vi "CreateInputTunnels.vi"(5 "controlling":bool, 6 "error in":errorcluster, 9 "Loop in":refnum<class "Loop.lvclass">) -> (0 "error out":errorcluster, 3 "Loop out":refnum<class "Loop.lvclass">, 4 "createTunnels":string)   [LabVIEW 2014, in "Raspberry Pi Compatible Compiler for LabVIEW.lvlib" / "Loop.lvclass"]
uses:
  Loop.lvclass
  Python/Parsing/ClassTypeTD.ctl
  Python/Parsing/ListTypesTD.ctl
  LoopTunnel/LoopTunnel.lvclass/LoopTunnel.ctl
  Tunnel/Tunnel.lvclass/Tunnel.ctl
  Terminal/Terminal.lvclass
  Python/Parsing/Python Functions.lvlib
  LoopTunnel/LoopTunnel.lvclass
  Tunnel/Tunnel.lvclass
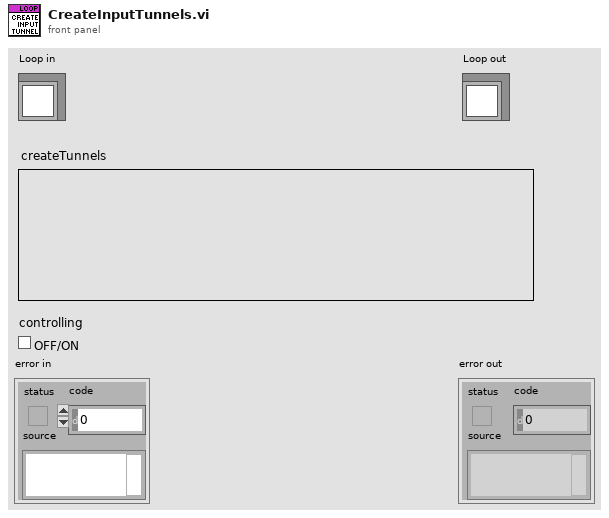
[diagram p1: front panel]
types:
  T1 = typedef "Raspberry Pi Compatible Compiler for LabVIEW.lvlib/Python Functions.lvlib/ListTypesTD.ctl" = enum16{"list", "tuple", "parameter list", "output list", "return values"}
  T2 = typedef "Raspberry Pi Compatible Compiler for LabVIEW.lvlib/Python Functions.lvlib/ClassTypeTD.ctl" = enum16{"class", "function"}
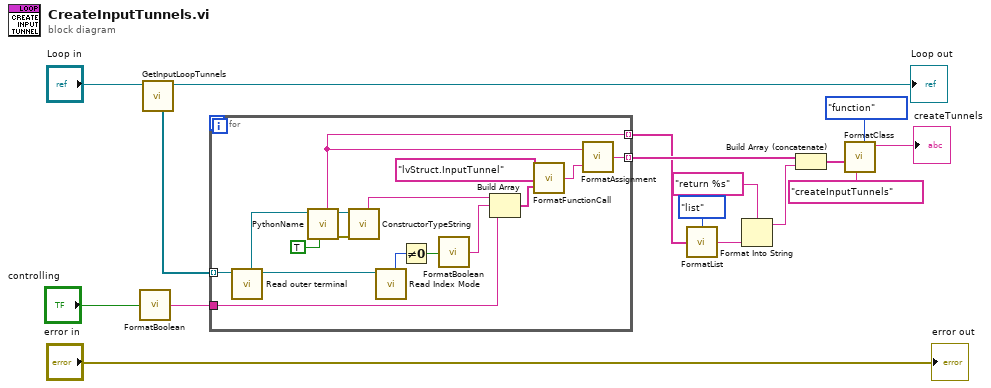
[diagram p0: block diagram]
diagram:
  n1 = call "FormatBoolean.vi"("value"="controlling") -> ("python object"=w7:string)
  n2 = call-dynamic "GetInputLoopTunnels.vi"("Loop in"="Loop in") -> ("Loop out"=→"Loop out":refnum<class "Loop.lvclass">, "tunnels"=w11:refnum<class "LoopTunnel.lvclass">[])  [unwired: 6 in, 1 out]
  n3 = for {
    tunnel: w11 -> [w30] mode=indexing
    tunnel: [w25] -> w10 mode=indexing
    tunnel: w7 -> [w19]
    tunnel: [w17] -> w6 mode=indexing
    n4 = call "Read outer terminal.vi"("Tunnel in"=w30) -> ("Tunnel out"=w31:refnum<class "LoopTunnel.lvclass">, "outer terminal"=w18:refnum<class "Terminal.lvclass">)  [unwired: 7 in]
    n5 = call-dynamic "PythonName.vi"("add self"=TRUE, "Terminal in"=w18) -> ("error out"=w28:errorcluster, "Terminal out"=w29:refnum<class "Terminal.lvclass">, "name"=w17:string)  [unwired: 6 in, 1 out]
    n6 = call "ConstructorTypeString.vi"("error in"=w28, "Terminal in"=w29) -> ("constructor string"=w22:string)  [unwired: 5 in, 2 out]
    n7 = call "Read Index Mode.vi"("LoopTunnel in"=w31) -> ("Index Mode"=w27:u32)  [unwired: 7 in, 1 out]
    n8 = Not Equal To 0?(x=w27) -> (x != 0?=w23:bool)
    n9 = call "FormatBoolean.vi"("value"=w23) -> ("python object"=w21:string)
    n10 = Build Array(w22, w21, w19) -> (w20:string[])
    n11 = call "FormatFunctionCall.vi"("parameters"=w20, "function"="lvStruct.InputTunnel" ("format string")) -> ("python object"=w24:string)
    n12 = call "FormatAssignment.vi"("value"=w24, "name"=w17) -> ("python assignment"=w25:string)
  }
  n13 = call "FormatList.vi"("values"=w6, "type"=ListTypesTD."list") -> ("python object"=w4:string)
  n14 = Format Into String(format string="return %s", w4) -> (resulting string=w1:string)  [unwired: 2 in, 1 out]
  n15 = Build Array (concatenate)(w10, w1) -> (w2:string[])
  n16 = call "FormatClass.vi"("type"=ClassTypeTD."function", "name"="createInputTunnels", "body"=w2) -> ("python"=→"createTunnels":string)  [unwired: 8 in]
  "error out" <- "error in"
